vi "Build Parameters.vi"(10 "Array in":cluster{"Scenario":string, "Parameters":T2}[](array[cluster])) -> (2 "Array out":T1(array[cluster]))   [LabVIEW 2020, in "Temperature Converter Test.lvclass"]
uses:
  Temperature Converter Test.lvclass
  Parameters.ctl
  Temperature Converter Test.lvclass/Temperature Converter Test.ctl
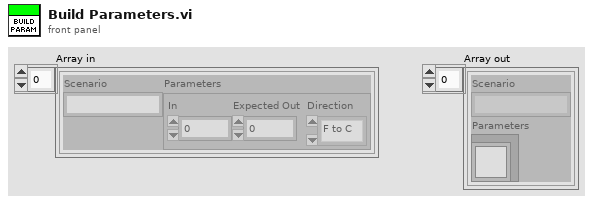
[diagram p1: front panel]
types:
  T1 = cluster{"Scenario":string, "Parameters":refnum<class "Temperature Converter Test.lvclass">}[]
  T2 = typedef "Temperature Converter Test.lvclass/Parameters.ctl" = cluster{"In":dbl, "Expected Out":dbl, "Direction":enum16{"F to C", "C to F"}}
  T3 = cluster{"Scenario":string, "Parameters":refnum<class "Temperature Converter Test.lvclass">}
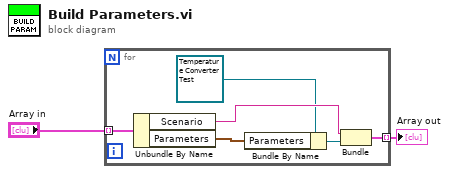
[diagram p0: block diagram]
diagram:
  n1 = for {
    tunnel: [w4] -> w1 mode=indexing
    tunnel: "Array in" -> [w8] mode=indexing
    n2 = Unbundle By Name(w8) -> ("Scenario"=w7:string, "Parameters"=w3:T2)
    n3 = Bundle By Name(cluster=refnum<class "Temperature Converter Test.lvclass"> refnum ("Parameters"), "Parameters"=w3) -> (w5:refnum<class "Temperature Converter Test.lvclass">)
    n4 = Bundle("Scenario"=w7, "Parameters"=w5) -> (w4:T3)  [unwired: 1 in]
  }
  "Array out" <- w1
